vi "Start Access Point.vi"(8 "Error In":errorcluster, 11 "EZ430-Chronos Ref":T1) -> (0 "Error Out":errorcluster, 3 "EZ430-Chronos Ref":T1)   [LabVIEW 2011, in "LVH-EZ430.lvlib"]
doc: "Start the access point in the user specified mode."
uses:
  LVH-EZ430.lvlib
  Type Defs/EZ430-Chronos Ref.ctl
  Type Defs/Command.ctl
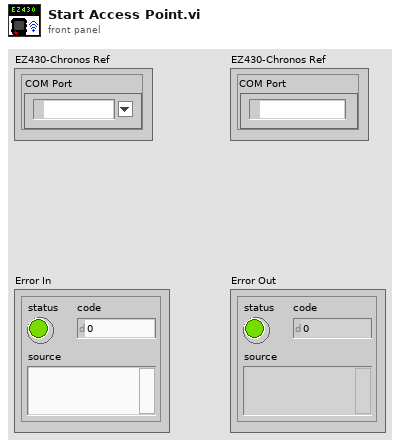
[diagram p1: front panel]
types:
  T1 = typedef "LVH-EZ430.lvlib/EZ430-Chronos Ref.ctl" = cluster{"COM Port":refnum<visa-resource-name>}
  T2 = typedef "LVH-EZ430.lvlib/Command.ctl" = enum8{"Get Hardware Status", "Reset RF Access Point", "Start BlueRobin Transmitter", "Set BlueRobin Trans ID", "Get BlueRobin Trans ID", "Set BlueRobin Heart Rate To Transmit", "Stop BlueRobin Transmitter", "Start ACC / PPT Mode", "Read ACC / PPT", "Stop SimpliciTI Stack"}
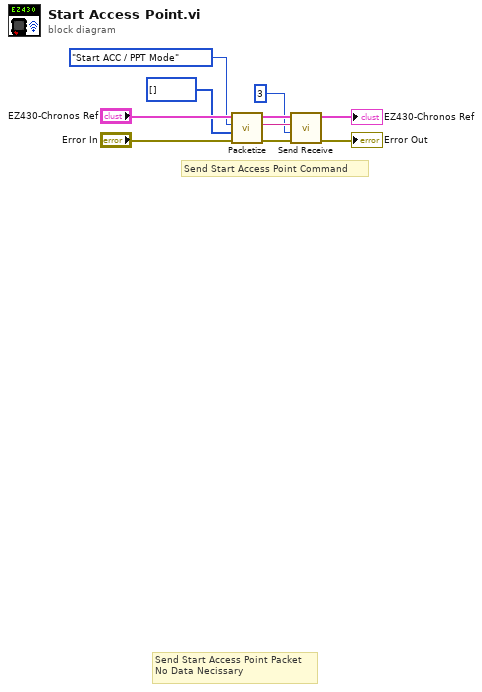
[diagram p0: block diagram]
diagram:
  # "Send Start Access Point Command"
  # "Send Start Access Point Packet\nNo Data Necissary"
  n1 = call "Packetize.vi"("Error In"="Error In", "Data"=u8[] [], "Command"=Command."Start ACC / PPT Mode", "EZ430-Chronos Config"="EZ430-Chronos Ref") -> ("Error Out"=w7:errorcluster, "Packet"=w5:string, "EZ430-Chronos Config"=w9:T1)  [unwired: 5 in]
  n2 = call "Send Receive.vi"("Error In"=w7, "Bytes To Read"=u32 3, "Packet"=w5, "EZ430-Chronos Config"=w9) -> ("Error Out"=→"Error Out":errorcluster, "EZ430-Chronos Config"=→"EZ430-Chronos Ref":T1)  [unwired: 5 in, 1 out]
